vi "ReadBoardInfo.vi"(10 "DeviceInd":u32, 11 "DeviceType":u32) -> (2 "VCI_BOARD_INFO":T1, 3 "success":bool)   [LabVIEW 2011]
uses:
  data/ControlCAN.dll
panel:
  out "VCI_BOARD_INFO_1":T2
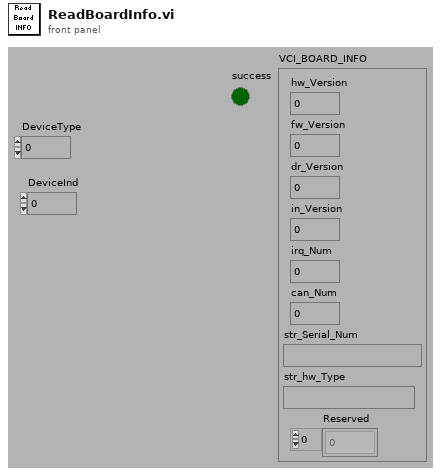
[diagram p1: front panel]
types:
  T1 = cluster{"hw_Version":u16, "fw_Version":u16, "dr_Version":u16, "in_Version":u16, "irq_Num":u16, "can_Num":u8, "str_Serial_Num":string, "str_hw_Type":string, "Reserved":u8[]}
  T2 = cluster{"hw_Version":u16, "fw_Version":u16, "dr_Version":u16, "in_Version":u16, "irq_Num":u16, "can_Num":u8, "str_Serial_Num 0":u8, "str_Serial_Num 1":u8, "str_Serial_Num 2":u8, "str_Serial_Num 3":u8, "str_Serial_Num 4":u8, "str_Serial_Num 5":u8, "str_Serial_Num 6":u8, "str_Serial_Num 7":u8, "str_Serial_Num 8":u8, "str_Serial_Num 9":u8, "str_Serial_Num 10":u8, "str_Serial_Num 11":u8, "str_Serial_Num 12":u8, "str_Serial_Num 13":u8, "str_Serial_Num 14":u8, "str_Serial_Num 15":u8, "str_Serial_Num 16":u8, "str_Serial_Num 17":u8, "str_Serial_Num 18":u8, "str_Serial_Num 19":u8, "str_hw_Type 0":u8, "str_hw_Type 1":u8, "str_hw_Type 2":u8, "str_hw_Type 3":u8, "str_hw_Type 4":u8, "str_hw_Type 5":u8, "str_hw_Type 6":u8, "str_hw_Type 7":u8, "str_hw_Type 8":u8, "str_hw_Type 9":u8, "str_hw_Type 10":u8, "str_hw_Type 11":u8, "str_hw_Type 12":u8, "str_hw_Type 13":u8, "str_hw_Type 14":u8, "str_hw_Type 15":u8, "str_hw_Type 16":u8, "str_hw_Type 17":u8, "str_hw_Type 18":u8, "str_hw_Type 19":u8, "str_hw_Type 20":u8, "str_hw_Type 21":u8, "str_hw_Type 22":u8, "str_hw_Type 24":u8, "str_hw_Type 25":u8, "str_hw_Type 26":u8, "str_hw_Type 27":u8, "str_hw_Type 28":u8, "str_hw_Type 29":u8, "str_hw_Type 30":u8, "str_hw_Type 31":u8, "str_hw_Type 32":u8, "str_hw_Type 33":u8, "str_hw_Type 34":u8, "str_hw_Type 35":u8, "str_hw_Type 36":u8, "str_hw_Type 37":u8, "str_hw_Type 38":u8, "str_hw_Type 39":u8, "Reserved 0":u8, "Reserved 1":u8, "Reserved 2":u8, "Reserved 3":u8}
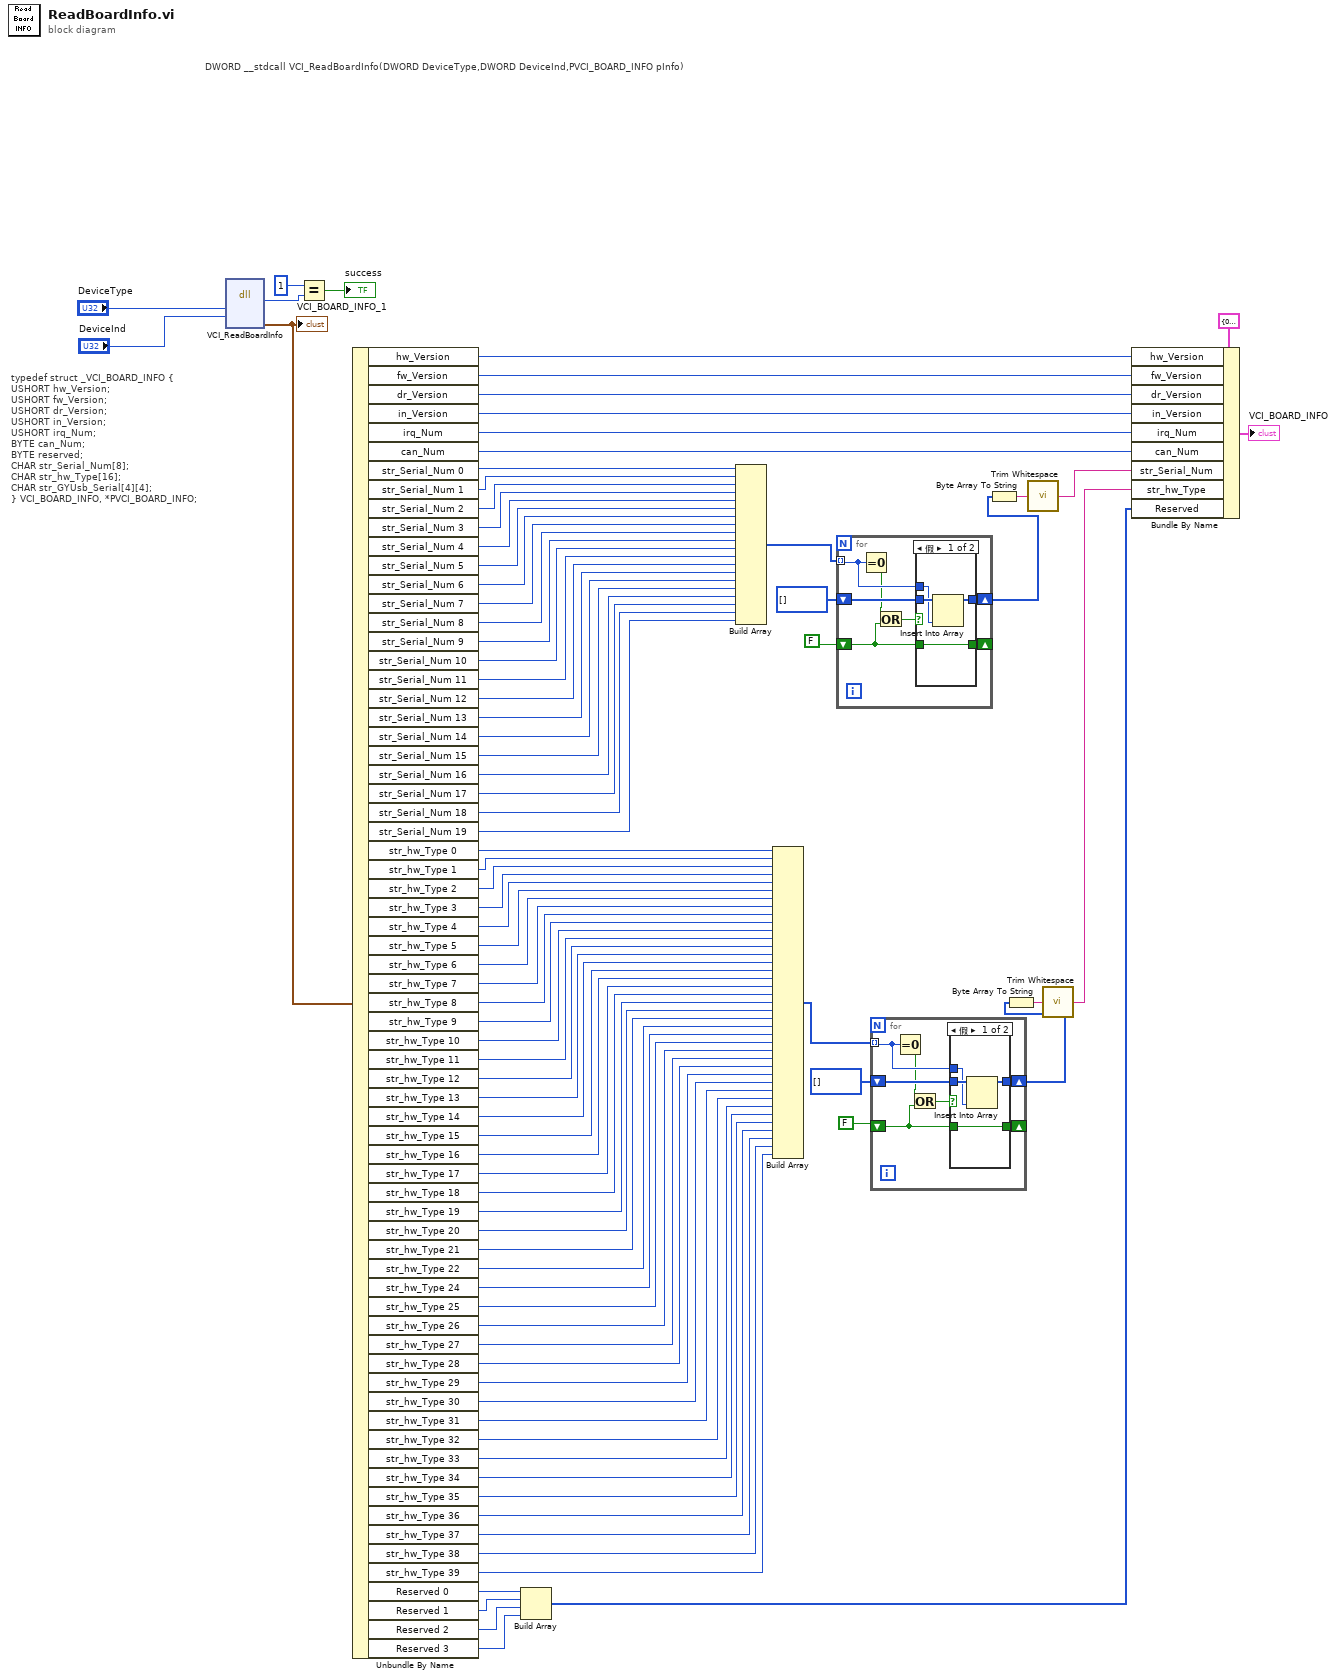
[diagram p0: block diagram]
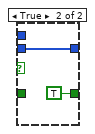
[diagram p2: hidden frame]
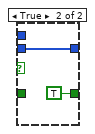
[diagram p3: hidden frame]
diagram:
  # "typedef struct _VCI_BOARD_INFO {\nUSHORT hw_Version;\nUSHORT fw_Version;\nUSHORT dr_Version;\nUSHORT in_Version;\nUSHORT irq_Num;\nBYTE can_Num;\nBYTE reserved;\nCHAR str_Serial_Num[8];\nCHAR str_hw_Type[16];\nCHAR str_GYUsb_Serial[4][4];\n} VCI_BOARD_INFO, *PVCI_BOARD_INFO;"
  # "DWORD __stdcall VCI_ReadBoardInfo(DWORD DeviceType,DWORD DeviceInd,PVCI_BOARD_INFO pInfo)"
  n1 = dll-call lib="PTH1vabs E工作USB-CAN Tool上位机源码USB-CAN Tool工具源码ZLG版USB CAN TooldataControlCAN.dll" fn="VCI_ReadBoardInfo" ("VCI_FindUsbDevice")("DeviceType"="DeviceType", "DeviceInd"="DeviceInd") -> ("返回类型"=w88:u32, "VCI_BOARD_INFO_1"=w10:T2)  [unwired: 6 in, 2 out]
  "VCI_BOARD_INFO_1" <- w10
  n2 = Equal?(x=u32 1, y=w88) -> (x = y?=→"success":bool)
  n3 = Unbundle By Name(w10) -> ("hw_Version"=w84:u16, "fw_Version"=w83:u16, "dr_Version"=w82:u16, "in_Version"=w81:u16, "irq_Num"=w80:u16, "can_Num"=w79:u8, "str_Serial_Num 0"=w78:u8, "str_Serial_Num 1"=w77:u8, "str_Serial_Num 2"=w76:u8, "str_Serial_Num 3"=w75:u8, "str_Serial_Num 4"=w74:u8, "str_Serial_Num 5"=w73:u8, "str_Serial_Num 6"=w72:u8, "str_Serial_Num 7"=w71:u8, "str_Serial_Num 8"=w68:u8, "str_Serial_Num 9"=w67:u8, "str_Serial_Num 10"=w66:u8, "str_Serial_Num 11"=w65:u8, "str_Serial_Num 12"=w64:u8, "str_Serial_Num 13"=w63:u8, "str_Serial_Num 14"=w62:u8, "str_Serial_Num 15"=w61:u8, "str_Serial_Num 16"=w60:u8, "str_Serial_Num 17"=w59:u8, "str_Serial_Num 18"=w58:u8, "str_Serial_Num 19"=w57:u8, "str_hw_Type 0"=w55:u8, "str_hw_Type 1"=w54:u8, "str_hw_Type 2"=w53:u8, "str_hw_Type 3"=w52:u8, "str_hw_Type 4"=w51:u8, "str_hw_Type 5"=w50:u8, "str_hw_Type 6"=w49:u8, "str_hw_Type 7"=w48:u8, "str_hw_Type 8"=w47:u8, "str_hw_Type 9"=w46:u8, "str_hw_Type 10"=w45:u8, "str_hw_Type 11"=w44:u8, "str_hw_Type 12"=w43:u8, "str_hw_Type 13"=w42:u8, "str_hw_Type 14"=w41:u8, "str_hw_Type 15"=w40:u8, "str_hw_Type 16"=w39:u8, "str_hw_Type 17"=w38:u8, "str_hw_Type 18"=w37:u8, "str_hw_Type 19"=w36:u8, "str_hw_Type 20"=w35:u8, "str_hw_Type 21"=w34:u8, "str_hw_Type 22"=w33:u8, "str_hw_Type 24"=w32:u8, "str_hw_Type 25"=w31:u8, "str_hw_Type 26"=w30:u8, "str_hw_Type 27"=w29:u8, "str_hw_Type 28"=w28:u8, "str_hw_Type 29"=w27:u8, "str_hw_Type 30"=w26:u8, "str_hw_Type 31"=w25:u8, "str_hw_Type 32"=w24:u8, "str_hw_Type 33"=w23:u8, "str_hw_Type 34"=w22:u8, "str_hw_Type 35"=w21:u8, "str_hw_Type 36"=w20:u8, "str_hw_Type 37"=w19:u8, "str_hw_Type 38"=w18:u8, "str_hw_Type 39"=w17:u8, "Reserved 0"=w16:u8, "Reserved 1"=w15:u8, "Reserved 2"=w14:u8, "Reserved 3"=w13:u8)
  n4 = Build Array(w16, w15, w14, w13) -> (w11:u8[])
  n5 = Build Array(w78, w77, w76, w75, w74, w73, w72, w71, w68, w67, w66, w65, w64, w63, w62, w61, w60, w59, w58, w57) -> (w2:u8[])
  n6 = Build Array(w55, w54, w53, w52, w51, w50, w49, w48, w47, w46, w45, w44, w43, w42, w41, w40, w39, w38, w37, w36, w35, w34, w33, w32, w31, w30, w29, w28, w27, w26, w25, w24, w23, w22, w21, w20, w19, w18, w17) -> (w6:u8[])
  n7 = for {
    tunnel: w2 -> [w97] mode=indexing
    shift-right: [w96] -> w1
    shift-left: u8[] [] -> [w95]
    shift-right: [w91] -> _
    shift-left: FALSE -> [w92]
    n8 = Equal To 0?(x=w97) -> (x = 0?=w94:bool)
    n9 = Or(x=w94, y=w92) -> (x .or. y?=w93:bool)
    n10 = case shown="假" w93 {
      tunnel: w97 -> [w100 _]
      tunnel: w95 -> [w101 w103]
      tunnel: [w99 w103] -> w96
      tunnel: w92 -> [w98 _]
      tunnel: [w98 TRUE] -> w91
      frame False {
        n11 = Insert Into Array(array=w101, new element=w100) -> (w99:u8[])  [unwired: 1 in]
      }
      frame True {
      }
    }
  }
  n12 = for {
    tunnel: w6 -> [w110] mode=indexing
    shift-right: [w109] -> w5
    shift-left: u8[] [] -> [w108]
    shift-right: [w104] -> _
    shift-left: FALSE -> [w105]
    n13 = Equal To 0?(x=w110) -> (x = 0?=w107:bool)
    n14 = Or(x=w107, y=w105) -> (x .or. y?=w106:bool)
    n15 = case shown="假" w106 {
      tunnel: w110 -> [w113 _]
      tunnel: w108 -> [w114 w116]
      tunnel: [w112 w116] -> w109
      tunnel: w105 -> [w111 _]
      tunnel: [w111 TRUE] -> w104
      frame False {
        n16 = Insert Into Array(array=w114, new element=w113) -> (w112:u8[])  [unwired: 1 in]
      }
      frame True {
      }
    }
  }
  n17 = Byte Array To String(unsigned byte array=w1) -> (string=w70:string)
  n18 = Byte Array To String(unsigned byte array=w5) -> (string=w56:string)
  n19 = call <vilib>:"Trim Whitespace.vi"("string"=w70) -> ("trimmed string"=w69:string)  [unwired: 1 in]
  n20 = call <vilib>:"Trim Whitespace.vi"("string"=w56) -> ("trimmed string"=w12:string)  [unwired: 1 in]
  n21 = Bundle By Name(cluster=T1 {"hw_Version"=0, "fw_Version"=0, "dr_Version"=0, "in_Version"=0, "irq_Num"=0, "can_Num"=0, "str_Serial_Num"="", "str_hw_Type"="", "Reserved"=[]} ("VCI_BOARD_INFO"), "hw_Version"=w84, "fw_Version"=w83, "dr_Version"=w82, "in_Version"=w81, "irq_Num"=w80, "can_Num"=w79, "str_Serial_Num"=w69, "str_hw_Type"=w12, "Reserved"=w11) -> (→"VCI_BOARD_INFO":T1)
